vi "3.3 Building Virtual Instruments-Lab1(Prob3).vi"() -> ()   [LabVIEW 2025]
panel:
  in  "stop":bool
  out "X < 0":bool
  out "X\nX = (A+B)*(C-1)":dbl
  in  "C":dbl
  in  "B":dbl
  in  "A":dbl
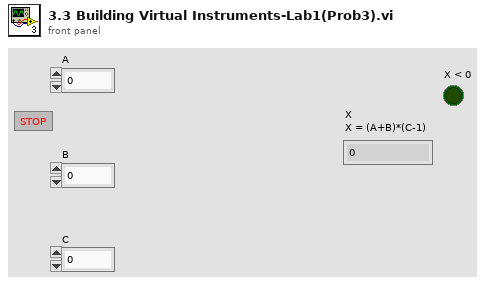
[diagram p1: front panel]
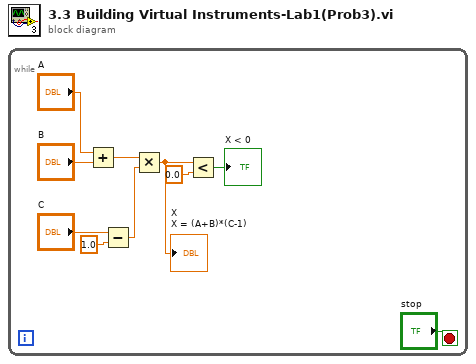
[diagram p0: block diagram]
diagram:
  n1 = while {
    stop <- "stop" stop-if-true
    n2 = Add(x="A", y="B") -> (x+y=w8:dbl)
    n3 = Subtract(x="C", y=1.0) -> (x-y=w5:dbl)
    n4 = Multiply(x=w8, y=w5) -> (x*y=w4:dbl)
    "X\nX = (A+B)*(C-1)" <- w4
    n5 = Less?(x=w4, y=0.0) -> (x < y?=→"X < 0":bool)
  }
